vi "Set Icon Template With VI Scope.vi"() -> ()   [LabVIEW 2020]
uses:
  <vilib>/LabVIEW Icon API/lv_icon/Classes/Icon Framework/Icon Framework.lvclass
  <vilib>/LabVIEW Icon API/lv_icon/Controls/Layer.ctl
  <vilib>/picture/picture.llb/imagedata.ctl
  <vilib>/LabVIEW Icon API/lv_icon/Classes/Layer/Layer.lvclass
  <vilib>/LabVIEW Icon API/lv_icon/Classes/Icon/Icon.lvclass
  <vilib>/LabVIEW Icon API/LabVIEW Icon API.lvlib
panel:
  in  "Nonexistent Project":bool
  in  "Class Path":path
  in  "Host":bool=TRUE
  in  "Project Path":path
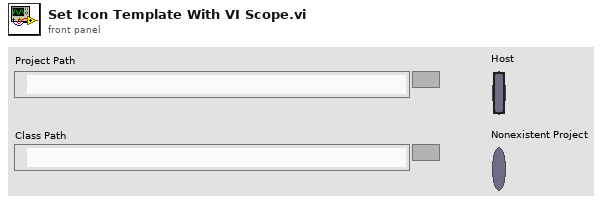
[diagram p1: front panel]
types:
  T1 = typedef "Layer.ctl" = cluster{"LayerIcon":picture, "LayerName":string, "Opacity":u8, "Visibility?":bool}
  T2 = enum32{"invalid scope", "public", "private", "protected", "community"}
  T3 = typedef "imagedata.ctl" = cluster{"image type":i32, "image depth":i32, "image":u8[], "mask":u8[], "colors":u32[], "Rectangle":cluster{"left":i16, "top":i16, "right":i16, "bottom":i16}}
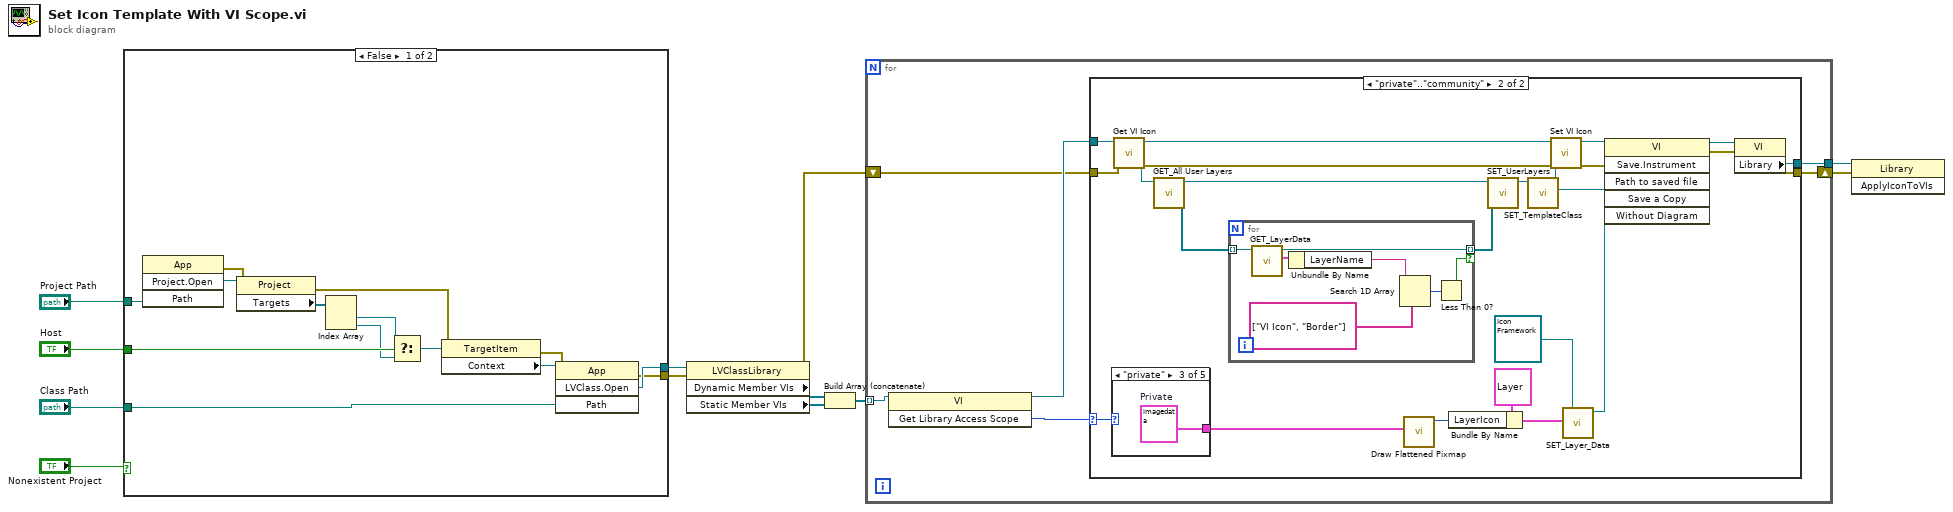
[diagram p0: block diagram]
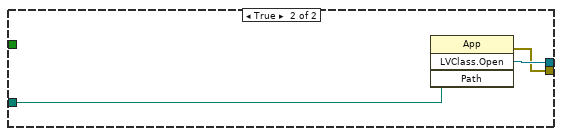
[diagram p2: hidden frame]
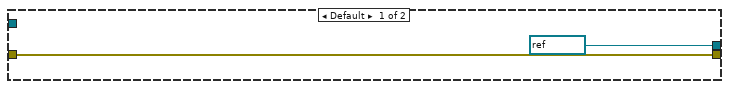
[diagram p3: hidden frame]
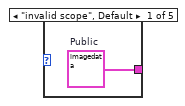
[diagram p4: hidden frame]
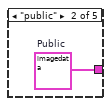
[diagram p5: hidden frame]
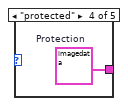
[diagram p6: hidden frame]
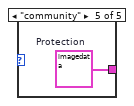
[diagram p7: hidden frame]
diagram:
  n1 = case shown="False" "Nonexistent Project" {
    tunnel: "Project Path" -> [w26 _]
    tunnel: "Host" -> [w23 _]
    tunnel: [w18 w29] -> w10
    tunnel: "Class Path" -> [w17 w28]
    tunnel: [w16 w27] -> w3
    frame False {
      n2 = invoke class="App" method="Project.Open"("Path"=w26) -> (error out=w13:errorcluster, "Project:Open"=w25:refnum<vi>)  [unwired: 3 in, 2 out]
      n3 = property class="Project"(reference=w25, error in=w13) -> (error out=w14:errorcluster, "Targets"=w24:refnum<vi>[])  [unwired: 1 out]
      n4 = Index Array(array=w24) -> (element #1=w22:refnum<vi>, element #2=w21:refnum<vi>)  [unwired: 2 in]
      n5 = Select(t=w22, s=w23, f=w21) -> (s? t:f=w20:refnum<vi>)
      n6 = property class="TargetItem"(reference=w20, error in=w14) -> (error out=w15:errorcluster, "Context"=w19:refnum<vi>)  [unwired: 1 out]
      n7 = invoke class="App" method="LVClass.Open"(reference=w19, error in=w15, "Path"=w17) -> (error out=w16:errorcluster, "LVClass.Open"=w18:refnum<vi>)  [unwired: 1 in, 2 out]
    }
    frame True {
      n8 = invoke class="App" method="LVClass.Open"("Path"=w28) -> (error out=w27:errorcluster, "LVClass.Open"=w29:refnum<vi>)  [unwired: 3 in, 2 out]
    }
  }
  n9 = property class="LVClassLibrary"(reference=w10, error in=w3) -> (error out=w1:errorcluster, "Dynamic Member VIs"=w9:refnum<vi>[], "Static Member VIs"=w8:refnum<vi>[])  [unwired: 1 out]
  n10 = Build Array (concatenate)(w9, w8) -> (w7:refnum<vi>[])
  n11 = for {
    tunnel: w7 -> [w35] mode=indexing
    tunnel: [w33] -> w6
    shift-right: [w31] -> w2
    shift-left: w1 -> [w30]
    n12 = invoke class="VI" method="Get Library Access Scope"(reference=w35) -> (reference out=w34:refnum<vi>, "Get Library Access Scope"=w32:T2)  [unwired: 2 in, 1 out]
    n13 = case shown="\"private\"..\"community\"" w32 {
      selector: w32 -> [_ w44]
      tunnel: w34 -> [_ w60]
      tunnel: [refnum<vi> refnum ("Library") w45] -> w33
      tunnel: [w36 w40] -> w31
      tunnel: w30 -> [w36 w39]
      frame Default {
      }
      frame "private".."community" {
        n14 = case shown="\"private\"" w44 {
          tunnel: [w61 w62 w63 w64 w65] -> w43
          frame "invalid scope", Default {
            w61 = T3 {"image type"=0, "image depth"=24, "image"=array[3072 elements], "mask"=[], "colors"=[], "Rectangle"={"left"=0, "top"=0, "right"=32, "bottom"=32}}  # Public
          }
          frame "public" {
            w62 = T3 {"image type"=0, "image depth"=24, "image"=array[3072 elements], "mask"=[], "colors"=[], "Rectangle"={"left"=0, "top"=0, "right"=32, "bottom"=32}}  # Public
          }
          frame "private" {
            w63 = T3 {"image type"=0, "image depth"=24, "image"=array[3072 elements], "mask"=[], "colors"=[], "Rectangle"={"left"=0, "top"=0, "right"=32, "bottom"=32}}  # Private
          }
          frame "protected" {
            w64 = T3 {"image type"=0, "image depth"=24, "image"=array[3072 elements], "mask"=[], "colors"=[], "Rectangle"={"left"=0, "top"=0, "right"=32, "bottom"=32}}  # Protection
          }
          frame "community" {
            w65 = T3 {"image type"=0, "image depth"=24, "image"=array[3072 elements], "mask"=[], "colors"=[], "Rectangle"={"left"=0, "top"=0, "right"=32, "bottom"=32}}  # Protection
          }
        }
        n15 = call <vilib>:"Get VI Icon.vi"("error in (no error)"=w39, "VI Refnum in"=w60) -> ("error out"=w38:errorcluster, "Icon"=w56:refnum<class "Icon.lvclass">, "VI Refnum out"=w59:refnum<vi>)  [unwired: 7 in]
        n16 = call-dynamic "GET_All User Layers.vi"("Icon.lvclass in"=w56) -> ("User Layer"=w55:refnum<class "Layer.lvclass">[], "Icon.lvclass out"=w58:refnum<class "Icon.lvclass">)  [unwired: 8 in, 1 out]
        n17 = for {
          tunnel: w55 -> [w72] mode=indexing
          tunnel: [w70] -> w57 mode=indexing if=w66
          n18 = call-dynamic "GET_LayerData.vi"("Layer.lvclass in"=w72) -> ("Data"=w71:T1, "Layer.lvclass out"=w70:refnum<class "Layer.lvclass">)  [unwired: 6 in, 3 out]
          n19 = Unbundle By Name(w71) -> ("LayerName"=w68:string)
          n20 = Search 1D Array(1D array=string[] ["VI Icon", "Border"], element=w68) -> (index of element=w67:i32)  [unwired: 1 in]
          n21 = Less Than 0?(x=w67) -> (x < 0?=w66:bool)
        }
        n22 = call <vilib>:"Draw Flattened Pixmap.vi"("image data"=w43) -> ("new picture"=w48:picture)  [unwired: 8 in]
        n23 = Bundle By Name(cluster=T1 {"LayerIcon"=bytes[3102], "LayerName"="Template", "Opacity"=100, "Visibility?"=TRUE} ("Data"), "LayerIcon"=w48) -> (w49:T1)
        n24 = call-dynamic "SET_UserLayers.vi"("Layers"=w57, "Icon.lvclass in"=w58) -> ("Icon.lvclass out"=w53:refnum<class "Icon.lvclass">)  [unwired: 8 in, 1 out]
        n25 = call-dynamic "SET_Layer_Data.vi"("Data"=w49, "Layer.lvclass in"=refnum<class "Icon Framework.lvclass"> refnum ("Icon Framework.lvclass")) -> ("Layer.lvclass out"=w51:refnum<class "Icon Framework.lvclass">)  [unwired: 8 in, 1 out]
        n26 = call-dynamic "SET_TemplateClass.vi"("Icon Framework.lvclass"=w51, "Icon.lvclass in"=w53) -> ("Icon.lvclass out"=w52:refnum<class "Icon.lvclass">)  [unwired: 8 in, 1 out]
        n27 = call <vilib>:"Set VI Icon.vi"("error in (no error)"=w38, "Icon"=w52, "VI Refnum in"=w59) -> ("error out"=w42:errorcluster, "VI Refnum out"=w47:refnum<vi>)  [unwired: 7 in]
        n28 = invoke class="VI" method="Save.Instrument"(reference=w47, error in=w42) -> (reference out=w46:refnum<vi>, error out=w41:errorcluster)  [unwired: 4 in, 4 out]
        n29 = property class="VI"(reference=w46, error in=w41) -> (error out=w40:errorcluster, "Library"=w45:refnum<vi>)  [unwired: 1 out]
      }
    }
  }
  n30 = invoke class="Library" method="ApplyIconToVIs"(reference=w6, error in=w2) -> ()  [unwired: 1 in, 3 out]
